vi "DAQmx.vi"(10 "AO Count(uSec)":u32=5, 11 "AI Count(uSec)":u32=5) -> ()   [LabVIEW 2019]
uses:
  <vilib>/eio/EIONode/EIONode.xnode
  <vilib>/rvi/eio/common/nirviEmuTemplateMethod_errors.vi
  <vilib>/rvi/DataTransferAndStorage/Container/XNode/niFpgaContainer.xnode
  <vilib>/rvi/interface/RandomDataEmulation/nirviRandomDataFpgaReadWriteTemplate.vi
  <vilib>/rvi/FIFO/Fifo_Resource/niFpgaFifoEmulationRefIn.vi
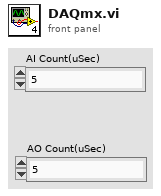
[diagram p1: front panel]
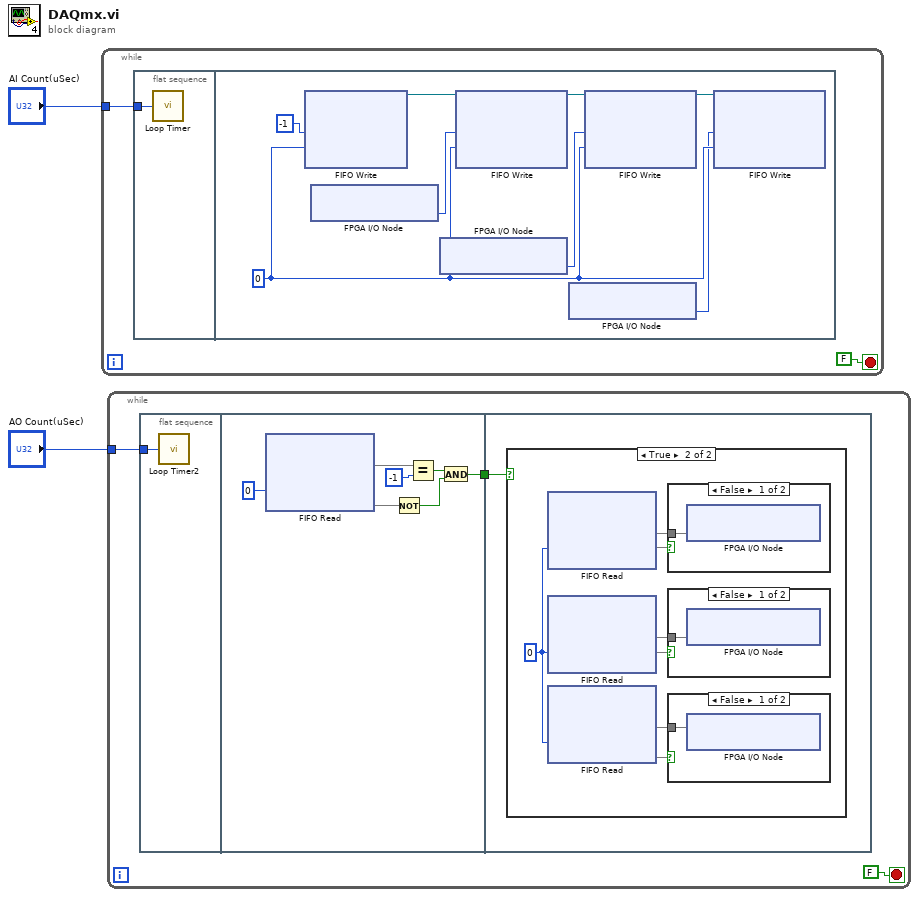
[diagram p0: block diagram]
diagram:
  n1 = while {
    tunnel: "AI Count(uSec)" -> [w3]
    stop <- FALSE stop-if-true
    n2 = flat-sequence {
      tunnel: w3 -> [w5]
      frame #0 {
        n3 = call "Loop Timer"("Count(uSec)"=w5) -> ()  [unwired: 1 out]
      }
      frame #1 {
        w10 = 0 ("Timeout")
        n4 = xnode ("FIFO Write")("Element"=i16 -1, "Timeout"=w10) -> ("FIFO Out"=w13:refnum<k21>)  [unwired: 1 in, 1 out]
        n5 = xnode "FPGA I/O Node"() -> ("Connector0/AI0"=w7:i16)  [unwired: 1 in, 1 out]
        n6 = xnode "FPGA I/O Node"() -> ("Connector0/AI1"=w8:i16)  [unwired: 1 in, 1 out]
        n7 = xnode ("FIFO Write")("Element"=w7, "Timeout"=w10, "FIFO In"=w13) -> ("FIFO Out"=w12:refnum<k21>)  [unwired: 1 out]
        n8 = xnode "FPGA I/O Node"() -> ("Connector0/AI2"=w9:i16)  [unwired: 1 in, 1 out]
        n9 = xnode ("FIFO Write")("Element"=w8, "Timeout"=w10, "FIFO In"=w12) -> ("FIFO Out"=w11:refnum<k21>)  [unwired: 1 out]
        n10 = xnode ("FIFO Write")("Element"=w9, "Timeout"=w10, "FIFO In"=w11) -> ()  [unwired: 2 out]
      }
    }
  }
  n11 = while {
    tunnel: "AO Count(uSec)" -> [w15]
    stop <- FALSE stop-if-true
    n12 = flat-sequence {
      tunnel: w15 -> [w17]
      tunnel: [w18] -> w14
      tunnel: w14 -> [w25]
      frame #0 {
        n13 = call "Loop Timer2"("Count(uSec)"=w17) -> ()  [unwired: 1 out]
      }
      frame #1 {
        n14 = xnode ("FIFO Read")("Timeout"=0) -> ("Element"=w23, "Timed Out?"=w20)  [unwired: 1 in, 1 out]
        n15 = Not(x=w20) -> (.not. x?=w19:bool)
        n16 = Equal?(x=w23, y=i16 -1) -> (x = y?=w21:bool)
        n17 = And(x=w21, y=w19) -> (x .and. y?=w18:bool)
      }
      frame #2 {
        n18 = case shown="True" w25 {
          frame False {
          }
          frame True {
            w28 = 0 ("Timeout")
            n19 = xnode ("FIFO Read")("Timeout"=w28) -> ("Element"=w32, "Timed Out?"=w31)  [unwired: 1 in, 1 out]
            n20 = xnode ("FIFO Read")("Timeout"=w28) -> ("Element"=w30, "Timed Out?"=w26)  [unwired: 1 in, 1 out]
            n21 = xnode ("FIFO Read")("Timeout"=w28) -> ("Element"=w29, "Timed Out?"=w27)  [unwired: 1 in, 1 out]
            n22 = case shown="False" w31 {
              tunnel: w32 -> [w35 _]
              frame False {
                n23 = xnode "FPGA I/O Node"("Connector0/AO0"=w35) -> ()  [unwired: 1 in, 1 out]
              }
              frame True {
              }
            }
            n24 = case shown="False" w26 {
              tunnel: w30 -> [w34 _]
              frame False {
                n25 = xnode "FPGA I/O Node"("Connector0/AO1"=w34) -> ()  [unwired: 1 in, 1 out]
              }
              frame True {
              }
            }
            n26 = case shown="False" w27 {
              tunnel: w29 -> [w33 _]
              frame False {
                n27 = xnode "FPGA I/O Node"("Connector0/AO2"=w33) -> ()  [unwired: 1 in, 1 out]
              }
              frame True {
              }
            }
          }
        }
      }
    }
  }
